vi "server.Server Data FGV.vi"(8 "error in (no error)":errorcluster, 10 "Action":enum16{"Initialize", "Check", "Close"}(ring)=enum."Check") -> (0 "error out":errorcluster, 1 "Responses Ref":refnum<data-value>, 3 "Request Queue":refnum<queue>, 4 "Server Running":bool)   [LabVIEW 2016, in "JSONRPC Server.lvclass"]
uses:
  JSONRPC Server.lvclass
  Request/Request.lvclass
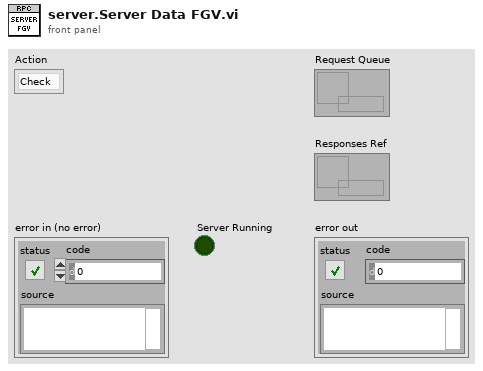
[diagram p1: front panel]
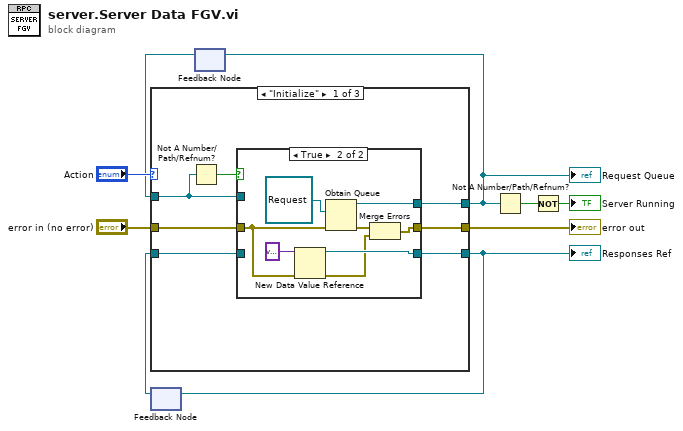
[diagram p0: block diagram]
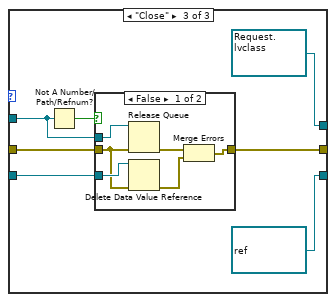
[diagram p4: hidden frame]
diagram:
  n1 = feedback #1() -> (w4:refnum<data-value>)  [unwired: 1 in]
  n2 = feedback #2() -> (w8:refnum<queue>)  [unwired: 1 in]
  n3 = case shown="\"Initialize\"" "Action" {
    tunnel: [w16 w29 refnum<queue> refnum ("queue out")] -> w3
    tunnel: w8 -> [w11 w29 w32]
    tunnel: "error in (no error)" -> [w15 w30 w35]
    tunnel: [w14 w30 w37] -> w6
    tunnel: [w13 w28 refnum<data-value> refnum ("data value reference")] -> w5
    tunnel: w4 -> [w12 w28 w36]
    frame "Initialize" {
      n4 = Not A Number/Path/Refnum?(number/path/refnum=w11) -> (NaN/Path/Refnum?=w10:bool)
      n5 = case shown="True" w10 {
        tunnel: [w18 w27] -> w16
        tunnel: w15 -> [w19 w20]
        tunnel: [w19 w24] -> w14
        tunnel: w11 -> [w18 _]
        tunnel: [w17 w22] -> w13
        tunnel: w12 -> [w17 _]
        frame False {
        }
        frame True {
          n6 = New Data Value Reference(data value=variant, error in=w20) -> (data value reference=w22:refnum<data-value>, error out=w21:errorcluster)
          n7 = Obtain Queue(element data type=refnum<class "Request.lvclass"> refnum ("Request.lvclass"), error in (no error)=w20) -> (queue out=w27:refnum<queue>, error out=w25:errorcluster)  [unwired: 3 in, 1 out]
          n8 = Merge Errors(w25, w21) -> (w24:errorcluster)
        }
      }
    }
    frame "Check" {
    }
    frame "Close" {
      n9 = Not A Number/Path/Refnum?(number/path/refnum=w32) -> (NaN/Path/Refnum?=w31:bool)
      n10 = case shown="False" w31 {
        tunnel: w32 -> [w43 _]
        tunnel: [w41 w44] -> w37
        tunnel: w36 -> [w40 _]
        tunnel: w35 -> [w38 w44]
        frame False {
          n11 = Release Queue(queue=w43, error in (no error)=w38) -> (error out=w42:errorcluster)  [unwired: 1 in, 2 out]
          n12 = Delete Data Value Reference(data value reference=w40, error in=w38) -> (error out=w39:errorcluster)  [unwired: 1 out]
          n13 = Merge Errors(w42, w39) -> (w41:errorcluster)
        }
        frame True {
        }
      }
    }
  }
  "error out" <- w6
  "Request Queue" <- w3
  "Responses Ref" <- w5
  n14 = feedback-in #1(w5) -> ()
  n15 = feedback-in #2(w3) -> ()
  n16 = Not A Number/Path/Refnum?(number/path/refnum=w3) -> (NaN/Path/Refnum?=w2:bool)
  n17 = Not(x=w2) -> (.not. x?=→"Server Running":bool)
